vi "PCO_SetROI.vi"(8 "error in (no error)":errorcluster, 9 "ROIend":cluster{"X":u16, "Y":u16}={"X"=1, "Y"=1}, 10 "ROIstart":cluster{"X":u16, "Y":u16}={"X"=1, "Y"=1}, 11 "Handle":u64) -> (0 "error out":errorcluster, 3 "Handle Out":u64, 5 "return type":u32 format="%x")   [LabVIEW 2011]
uses:
  SC2_Cam64.dll
panel:
  # "A00A3002 invalid Handle"
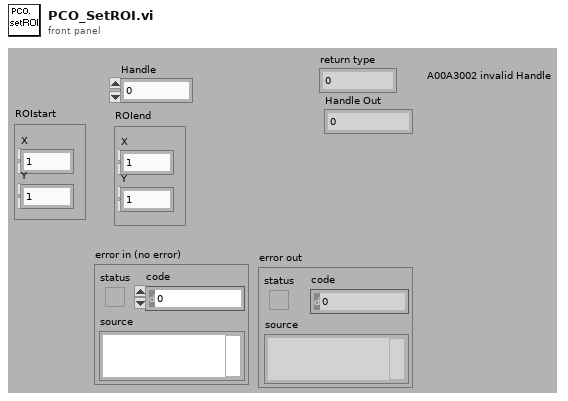
[diagram p1: front panel]
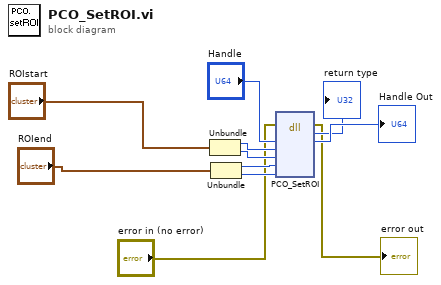
[diagram p0: block diagram]
diagram:
  n1 = Unbundle("ROIstart") -> ("X"=w6:u16, "Y"=w5:u16)
  n2 = Unbundle("ROIend") -> ("X"=w4:u16, "Y"=w3:u16)
  n3 = dll-call lib="C:/Program Files/colibri/Drivers/PCO.Camera/SC2_Cam*.*" fn="PCO_SetROI"(error in="error in (no error)", "Handle"="Handle", "wXResAct"=w6, "wYResAct"=w5, "wXResMax"=w4, "wYResMax"=w3) -> (error out=→"error out":errorcluster, "return type"=→"return type":u32, "Handle"=→"Handle Out":u64)  [unwired: 6 in, 1 out]
